vi "Close MeasurementLink Session.vi"(8 "error in (no error)":errorcluster, 9 "close session behavior":T1, 10 "session in":variant, 11 "instrument in":refnum<class "Fake Instrument.lvclass">) -> (0 "error out":errorcluster)   [LabVIEW 2020, in "MeasurementServerTests.lvlib" / "Fake Instrument.lvclass"]
doc: "Closes the local session. If the session represents a remote session, <b>close session behavior</b> determines whether closing the local session closes the server session or detaches from the server session."
uses:
  Fake Instrument.lvclass
  Runtime/MeasurementLink Instrument/IInstrument/Close Session Behavior.ctl
  Fake Instrument.lvclass/Fake Instrument.ctl
  Runtime/MeasurementLink Instrument/IInstrument/IInstrument.lvclass
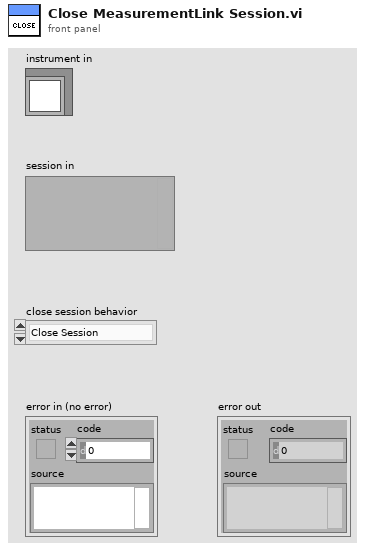
[diagram p1: front panel]
types:
  T1 = typedef "MeasurementLink Instrument.lvlib/IInstrument.lvclass/Close Session Behavior.ctl" = enum16{"Close Session", "Detach Session"}
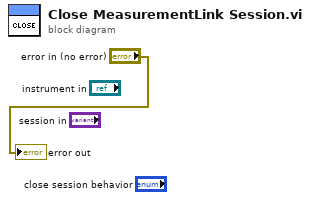
[diagram p0: block diagram]
diagram:
  "error out" <- "error in (no error)"
